vi "basic_Angle Rotate.vi"(11 "array in":cdb[](array[numeric])) -> (3 "array out":cdb[](array[numeric]))   [LabVIEW 2011, in "NI_EP_Basic.lvlib"]
doc: "The phase will modified according to the the first channel."
uses:
  <vilib>/addons/Electrical Power/Basic/NI_EP_Basic.lvlib
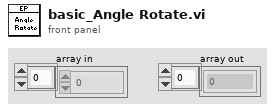
[diagram p1: front panel]
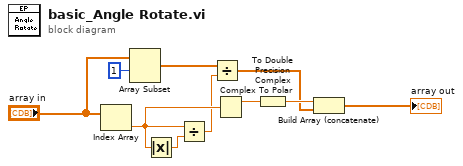
[diagram p0: block diagram]
diagram:
  n1 = Index Array(array="array in") -> (element=w6:cdb)  [unwired: 1 in]
  n2 = Array Subset(array="array in", index=1) -> (w4:cdb[])  [unwired: 1 in]
  n3 = Absolute Value(x=w6) -> (abs(x)=w3:dbl)
  n4 = Divide(x=w6, y=w3) -> (x/y=w5:cdb)
  n5 = Divide(x=w4, y=w5) -> (x/y=w8:cdb[])
  n6 = Complex To Polar(r * e^(i*theta)=w6) -> (r=w7:dbl)  [unwired: 1 out]
  n7 = To Double Precision Complex(1:w7) -> (0:w9:cdb)
  n8 = Build Array (concatenate)(w9, w8) -> (→"array out":cdb[])
